vi "perform fault handling.vi"(0 "module in":refnum<class "TBM module execution interface.lvclass">, 1 "module ref in":refnum<data-value>, 3 "error in":errorcluster, 4 "fault handling in":T4, 5 "run flags in":u8, 7 "engine error in":errorcluster, 8 "worker pool in":T1, 9 "cfg ref":refnum<data-value>, 11 "engine reference":i32, 12 "iteration":u64) -> (13 "engine error out":errorcluster, 14 "module out":refnum<class "TBM module execution interface.lvclass">, 15 "go to safe state":bool, 17 "error out":errorcluster, 19 "run flags out":u8)   [LabVIEW 2013, in "main engine.lvlib"]
doc: "Performs error handling actions for synchronous modules."
uses:
  main engine.lvlib
  fault handling spec.ctl
  Configuration/Error Actions.ctl
  <vilib>/NI/DCAF Module Framework/runtime/TBM module execution interface.lvclass
  worker library/worker comms.ctl
  worker library/worker commands.ctl
  worker library/request fifos.ctl
  worker library/recovery request.ctl
  <vilib>/NI/DCAF Module Framework/module configuration/TBM module configuration.lvclass
  worker library/rt fault.ctl
  <vilib>/NI/DCAF Module Framework/runtime/error classification.ctl
  worker library/response fifos.ctl
  worker library/recovery response.ctl
  <vilib>/NI/DCAF Execution Engine Interface/Engine Runtime/Fault.ctl
  worker library/worker pool.lvlib
  Configuration/Standard Engine Configuration.lvclass
  <vilib>/NI/DCAF Execution Engine Interface/Engine Runtime/Engine Runtime Interface.lvclass
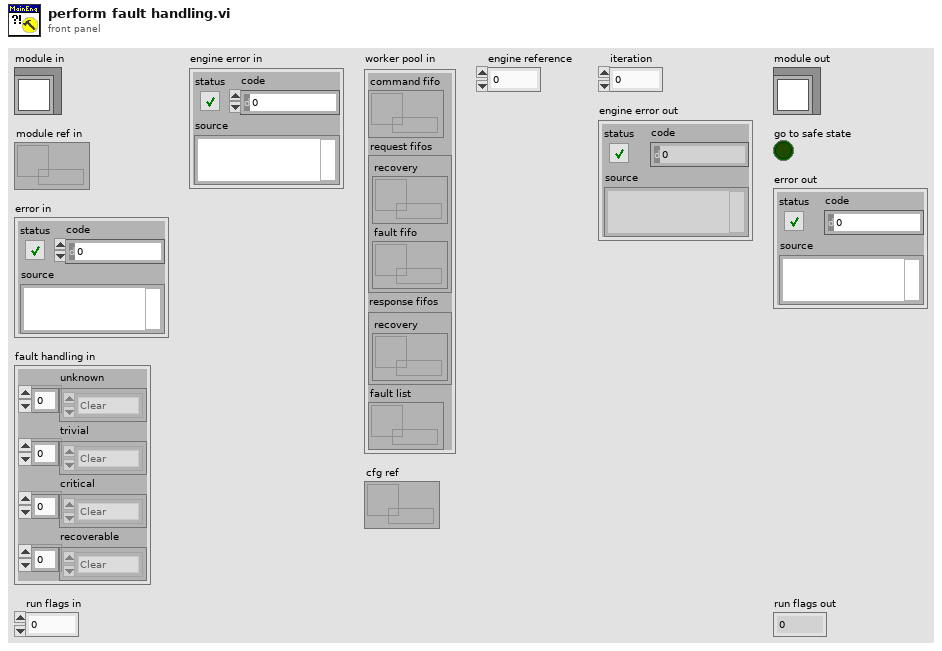
[diagram p1: front panel]
types:
  T1 = typedef "worker pool.lvlib/worker comms.ctl" = cluster{"command fifo":refnum<k33>, "request fifos":T2, "response fifos":T3, "fault list":refnum<data-value>}
  T2 = typedef "worker pool.lvlib/request fifos.ctl" = cluster{"recovery":refnum<k33>, "fault fifo":refnum<k33>}
  T3 = typedef "worker pool.lvlib/response fifos.ctl" = cluster{"recovery":refnum<k33>}
  T4 = typedef "main engine.lvlib/fault handling spec.ctl" = cluster{"unknown":T5[], "trivial":T5[], "critical":T5[], "recoverable":T5[]}
  T5 = typedef "Standard Engine Configuration.lvclass/Error Actions.ctl" = enum16{"Clear", "Notify", "Stop Component", "Stop Engine", "Safe State", "Attempt Recovery"}
  T6 = typedef "TBM module execution interface.lvclass/error classification.ctl" = enum16{"unknown", "none", "trivial", "recoverable", "critical"}
  T7 = typedef "worker pool.lvlib/rt fault.ctl" = cluster{"code":i32, "classification":T6, "iteration":u64, "cfg ref":refnum<data-value>}
  T8 = typedef "worker pool.lvlib/recovery request.ctl" = cluster{"module ref":refnum<data-value>, "engine reference":i32, "original run flags":u8, "attempts allowed":u16, "cfg ref":refnum<data-value>}
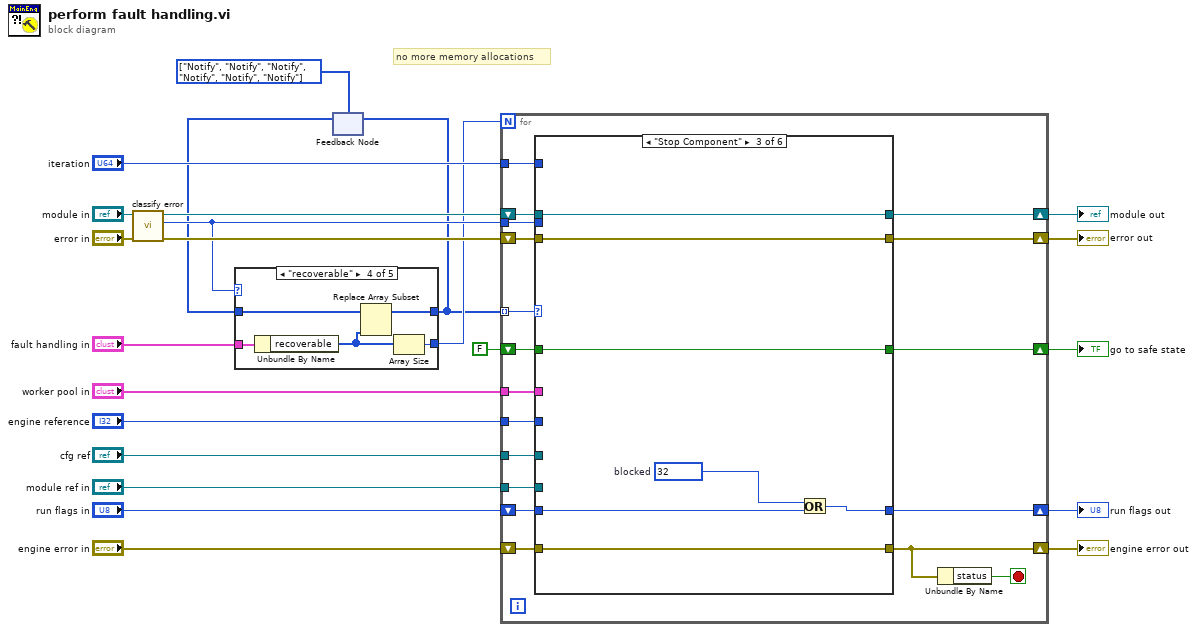
[diagram p0: block diagram]
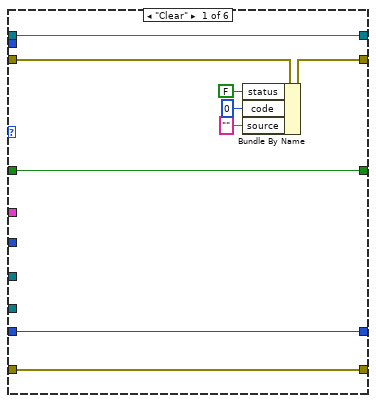
[diagram p2: hidden frame]
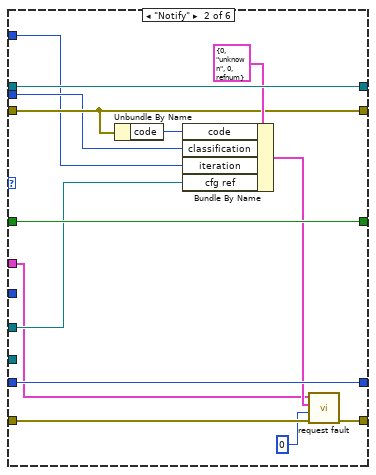
[diagram p3: hidden frame]
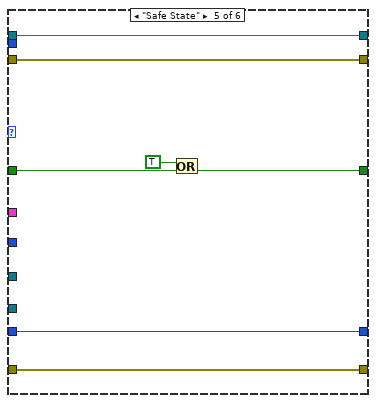
[diagram p5: hidden frame]
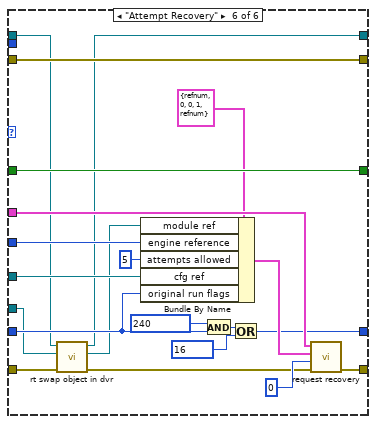
[diagram p6: hidden frame]
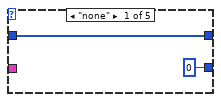
[diagram p7: hidden frame]
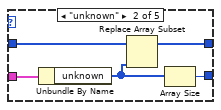
[diagram p8: hidden frame]
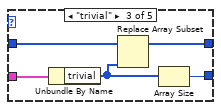
[diagram p9: hidden frame]
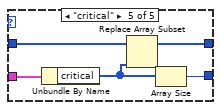
[diagram p10: hidden frame]
diagram:
  w1 = T5[] [enum."Notify", enum."Notify", enum."Notify", enum."Notify", enum."Notify", enum."Notify"] items=["Clear", "Notify", "Stop Component", "Stop Engine", "Safe State", "Attempt Recovery"] ("critical")
  # "no more memory allocations"
  n1 = call-dynamic "classify error.vi"("error to classify"="error in", "module in"="module in") -> ("classified error"=w18:errorcluster, "error classification"=w11:T6, "module out"=w17:refnum<class "TBM module execution interface.lvclass">)  [unwired: 7 in]
  n2 = feedback #1(w1) -> (w2:T5[])
  n3 = case shown="\"recoverable\"" w11 {
    tunnel: "fault handling in" -> [_ w30 w35 w40 w45]
    tunnel: [w24 w27 w32 w37 w42] -> w3
    tunnel: [0 w29 w34 w39 w44] -> w4
    tunnel: w2 -> [w24 w28 w33 w38 w43]
    frame "none" {
    }
    frame "unknown" {
      n4 = Unbundle By Name(w30) -> ("unknown"=w26:T5[])
      n5 = Replace Array Subset(array=w28, new element=w26) -> (w27:T5[])  [unwired: 1 in]
      n6 = Array Size(array=w26) -> (size(s)=w29:i32)
    }
    frame "trivial" {
      n7 = Unbundle By Name(w35) -> ("trivial"=w31:T5[])
      n8 = Replace Array Subset(array=w33, new element=w31) -> (w32:T5[])  [unwired: 1 in]
      n9 = Array Size(array=w31) -> (size(s)=w34:i32)
    }
    frame "recoverable" {
      n10 = Unbundle By Name(w40) -> ("recoverable"=w36:T5[])
      n11 = Replace Array Subset(array=w38, new element=w36) -> (w37:T5[])  [unwired: 1 in]
      n12 = Array Size(array=w36) -> (size(s)=w39:i32)
    }
    frame "critical" {
      n13 = Unbundle By Name(w45) -> ("critical"=w41:T5[])
      n14 = Replace Array Subset(array=w43, new element=w41) -> (w42:T5[])  [unwired: 1 in]
      n15 = Array Size(array=w41) -> (size(s)=w44:i32)
    }
  }
  n16 = feedback-in #1(w3) -> ()
  n17 = for {
    N: w4 -> [_]
    shift-right: [w56] -> w14
    shift-left: "run flags in" -> [w57]
    shift-right: [w59] -> w16
    shift-left: w18 -> [w60]
    shift-right: [w62] -> w15
    shift-left: w17 -> [w61]
    tunnel: w3 -> [w63] mode=indexing
    shift-right: [w54] -> w12
    shift-left: "engine error in" -> [w55]
    tunnel: w11 -> [w53]
    tunnel: "iteration" -> [w52]
    shift-right: [w51] -> w8
    shift-left: FALSE -> [w50]
    tunnel: "worker pool in" -> [w49]
    tunnel: "cfg ref" -> [w48]
    tunnel: "module ref in" -> [w58]
    tunnel: "engine reference" -> [w47]
    stop <- w46 stop-if-true
    n18 = case shown="\"Stop Component\"" w63 {
      tunnel: [w72 w86 w93 w97 w104 w107] -> w62
      tunnel: w61 -> [w72 w86 w93 w97 w104 w108]
      tunnel: w60 -> [w71 w83 w92 w95 w103 w125]
      tunnel: [w68 w83 w92 w95 w103 w125] -> w59
      tunnel: w58 -> [_ _ _ _ _ w110]
      tunnel: w57 -> [w70 w85 w89 w96 w102 w113]
      tunnel: [w70 w85 w88 w96 w102 w116] -> w56
      tunnel: w55 -> [w69 w76 w91 _ w101 w106]
      tunnel: [w69 w77 w91 w95 w101 w122] -> w54
      tunnel: w53 -> [_ w81 _ _ _ _]
      tunnel: w52 -> [_ w80 _ _ _ _]
      tunnel: [w64 w79 w90 w94 w99 w124] -> w51
      tunnel: w50 -> [w64 w79 w90 w94 w100 w124]
      tunnel: w49 -> [_ w74 _ _ _ w123]
      tunnel: w48 -> [_ w78 _ _ _ w112]
      tunnel: w47 -> [_ _ _ _ _ w114]
      frame "Clear" {
        n19 = Bundle By Name(cluster=w71, "status"=FALSE, "code"=0, "source"="") -> (w68:errorcluster)
      }
      frame "Notify" {
        n20 = Unbundle By Name(w83) -> ("code"=w82:i32)
        n21 = Bundle By Name(cluster=T7 {"code"=0, "classification"=enum."unknown", "iteration"=0, "cfg ref"=refnum} ("element"), "code"=w82, "classification"=w81, "iteration"=w80, "cfg ref"=w78) -> (w75:T7)
        n22 = call "request fault.vi"("error in"=w76, "timeout in ms (0)"=0, "rt fault"=w75, "worker comms in"=w74) -> ("error out"=w77:errorcluster)  [unwired: 7 in]
      }
      frame "Stop Component" {
        w87 = u8 32  # blocked
        n23 = Or(x=w87, y=w89) -> (x .or. y?=w88:u8)
      }
      frame "Stop Engine" {
        # "Passing an engine error out stops the engine."
      }
      frame "Safe State" {
        n24 = Or(x=TRUE, y=w100) -> (x .or. y?=w99:bool)
      }
      frame "Attempt Recovery" {
        n25 = call "rt swap object in dvr.vi"("error in"=w106, "module ref in in"=w110, "module in"=w108) -> ("error out"=w105:errorcluster, "module ref out"=w109:refnum<data-value>, "module out"=w107:refnum<class "TBM module execution interface.lvclass">)  [unwired: 6 in]
        n26 = Bundle By Name(cluster=T8 {"module ref"=refnum, "engine reference"=0, "original run flags"=0, "attempts allowed"=1, "cfg ref"=refnum} ("recovery request"), "module ref"=w109, "engine reference"=w114, "attempts allowed"=u16 5, "cfg ref"=w112, "original run flags"=w113) -> (w119:T8)
        n27 = And(x=u8 240, y=w113) -> (x .and. y?=w118:u8)
        n28 = Or(x=w118, y=u8 16 ("x")) -> (x .or. y?=w116:u8)
        n29 = call "request recovery.vi"("error in"=w105, "timeout in ms (0)"=0, "recovery request"=w119, "worker comms in"=w123) -> ("error out"=w122:errorcluster)  [unwired: 7 in]
      }
    }
    n30 = Unbundle By Name(w54) -> ("status"=w46:bool)
  }
  "error out" <- w16
  "module out" <- w15
  "run flags out" <- w14
  "engine error out" <- w12
  "go to safe state" <- w8
